vi "cooling.vi"() -> ()   [LabVIEW 2015]
panel:
  out "Output file path":path
  in  "Thick_max":bool[](array[boolean])=[FALSE, FALSE, FALSE, FALSE, FALSE, FALSE, FALSE, FALSE, FALSE, FALSE]
  in  "Thick_min":bool[](array[boolean])=[FALSE, FALSE, FALSE, FALSE, FALSE, FALSE, FALSE, FALSE, FALSE, FALSE]
  in  "Wid_max":bool[](array[boolean])=[FALSE, FALSE, FALSE, FALSE, FALSE, FALSE, FALSE, FALSE, FALSE, FALSE]
  in  "Apri database":bool
  in  "Insert IDs":bool
  in  "Stop Button":bool
  in  "Refresh Button":bool
  in  "Crea file di testo":bool
  in  "Wid_min":bool[](array[boolean])=[FALSE, FALSE, FALSE, FALSE, FALSE, FALSE, FALSE, FALSE, FALSE, FALSE]
  out "Bar name":string[](array[string])
  # "Cooling \"go - no go\" test"
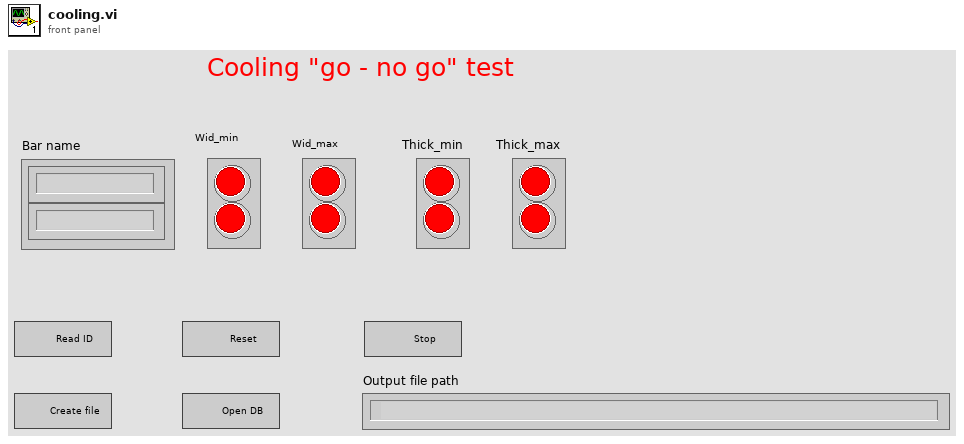
[diagram p1: front panel]
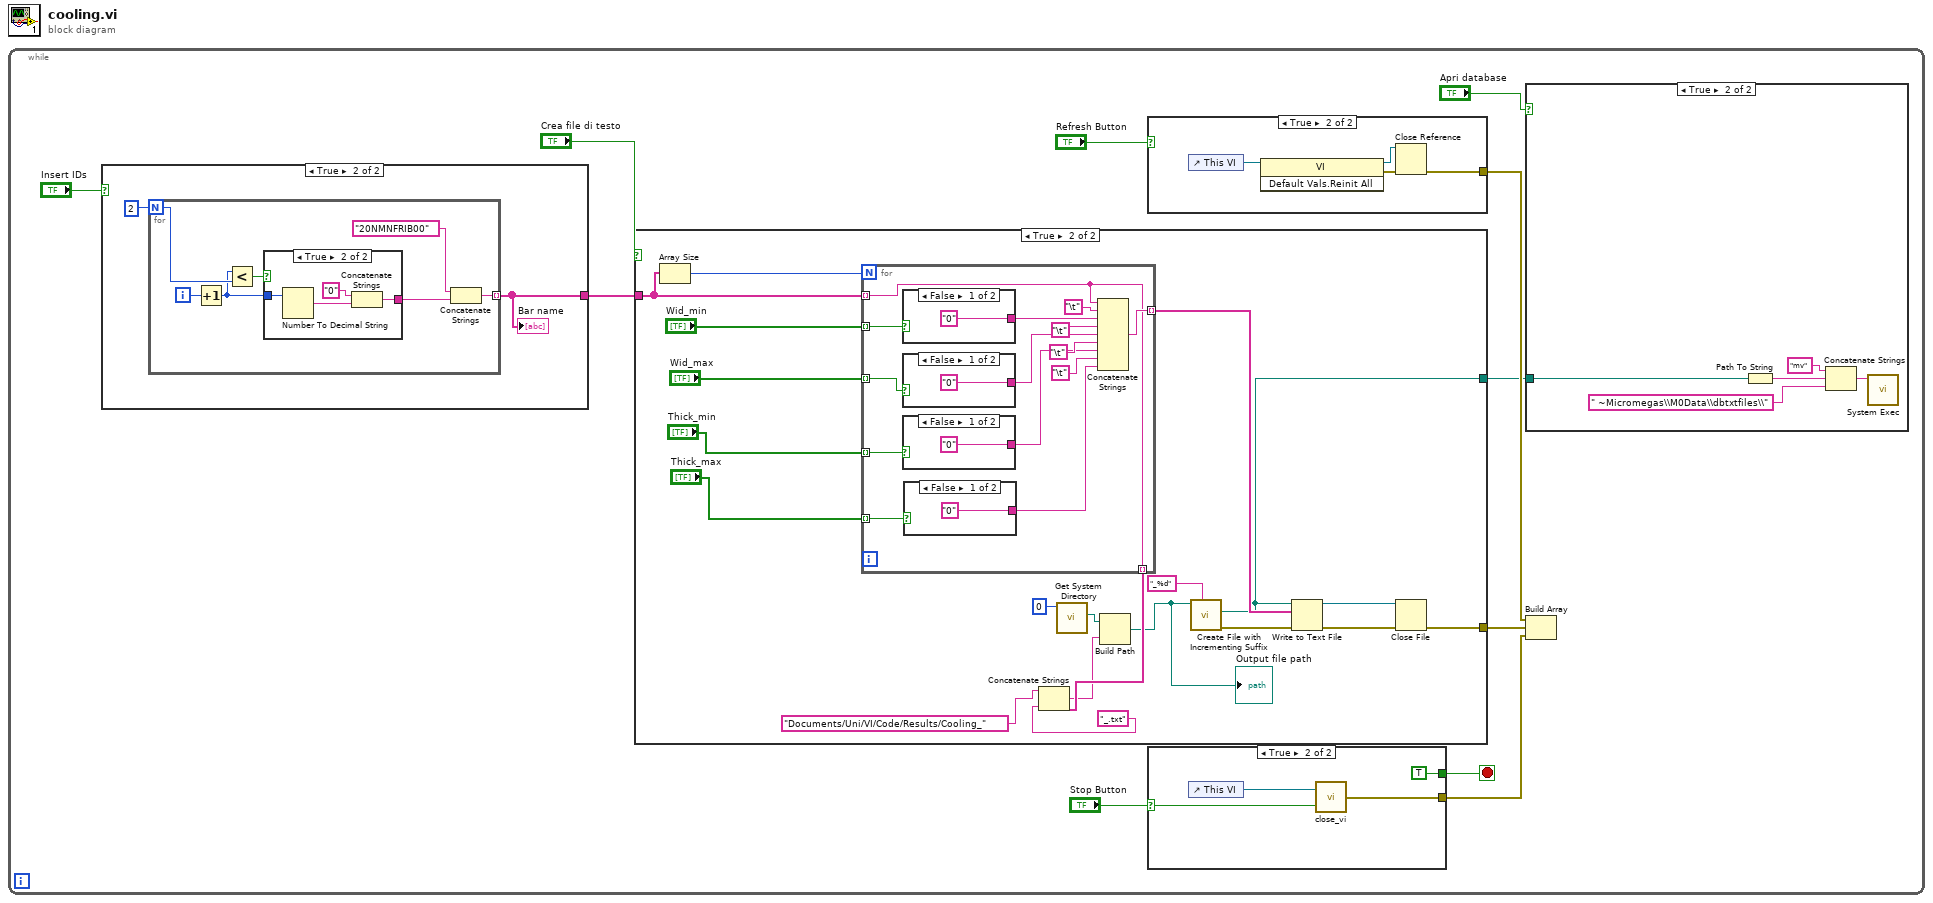
[diagram p0: block diagram]
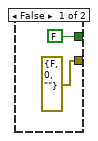
[diagram p3: hidden frame]
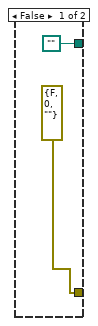
[diagram p4: hidden frame]
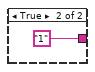
[diagram p5: hidden frame]
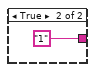
[diagram p6: hidden frame]
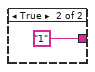
[diagram p7: hidden frame]
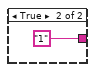
[diagram p8: hidden frame]
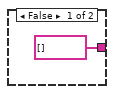
[diagram p9: hidden frame]
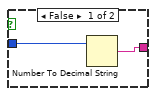
[diagram p10: hidden frame]
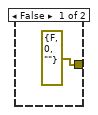
[diagram p11: hidden frame]
diagram:
  n1 = while {
    stop <- w3 stop-if-true
    n2 = case shown="True" "Insert IDs" {
      tunnel: [string[] [] w68] -> w8
      frame False {
      }
      frame True {
        n3 = for {
          N: 2 -> [w75]
          tunnel: [w70] -> w68 mode=indexing
          i -> [w74]
          n4 = Increment(x=w74) -> (x+1=w72:i32)
          n5 = Less?(x=w72, y=w75) -> (x < y?=w76:bool)
          n6 = case shown="True" w76 {
            tunnel: w72 -> [w78 w81]
            tunnel: [w77 w79] -> w71
            frame False {
              n7 = Number To Decimal String(number=w78) -> (decimal integer string=w77:string)  [unwired: 1 in]
            }
            frame True {
              n8 = Number To Decimal String(number=w81) -> (decimal integer string=w80:string)  [unwired: 1 in]
              n9 = Concatenate Strings("0", w80) -> (w79:string)
            }
          }
          n10 = Concatenate Strings("20NMNFRIB00", w71) -> (w70:string)
        }
        "Bar name" <- w68
      }
    }
    n11 = case shown="True" "Crea file di testo" {
      tunnel: w8 -> [_ w43]
      tunnel: [errorcluster {"status"=FALSE, "code"=0, "source"=""} ("error out") w36] -> w7
      tunnel: [path "" ("actual path") w35] -> w1
      frame False {
      }
      frame True {
        n12 = Array Size(array=w43) -> (size(s)=w44:i32)
        n13 = for {
          N: w44 -> [_]
          tunnel: w43 -> [w45] mode=indexing
          tunnel: "Wid_min" -> [w58] mode=indexing
          tunnel: [w55] -> w41 mode=indexing
          tunnel: "Wid_max" -> [w54] mode=indexing
          tunnel: "Thick_min" -> [w53] mode=indexing
          tunnel: "Thick_max" -> [w52] mode=indexing
          tunnel: [w45] -> w28 mode=indexing
          n14 = case shown="False" w58 {
            tunnel: ["0" "1"] -> w56
            frame False {
            }
            frame True {
            }
          }
          n15 = case shown="False" w54 {
            tunnel: ["0" "1"] -> w50
            frame False {
            }
            frame True {
            }
          }
          n16 = case shown="False" w53 {
            tunnel: ["0" "1"] -> w48
            frame False {
            }
            frame True {
            }
          }
          n17 = case shown="False" w52 {
            tunnel: ["0" "1"] -> w46
            frame False {
            }
            frame True {
            }
          }
          n18 = Concatenate Strings(w45, "\t", w56, "\t", w50, "\t", w48, "\t", w46) -> (w55:string)
        }
        n19 = Concatenate Strings("Documents/Uni/VI/Code/Results/Cooling_", w28, "_.txt") -> (w27:string)
        n20 = call <vilib>:"Get System Directory.vi"("system directory type"=0) -> ("system directory"=w30:path)  [unwired: 10 in]
        n21 = Build Path(base path=w30, name or relative path=w27) -> (appended path=w25:path)
        "Output file path" <- w25
        n22 = call <vilib>:"Create File with Incrementing Suffix.vi"("format string (\" (%d)\")"="_%d" ("format string (\" (%d)\")"), "file path"=w25) -> ("error out"=w40:errorcluster, "actual path"=w35:path)  [unwired: 7 in, 1 out]
        n23 = Write to Text File(file (use dialog)=w35, text=w41, error in=w40) -> (refnum out=w38:refnum<file>, error out=w39:errorcluster)  [unwired: 1 in, 1 out]
        n24 = Close File(refnum=w38, error in=w39) -> (error out=w36:errorcluster)  [unwired: 1 out]
      }
    }
    n25 = case shown="True" "Refresh Button" {
      tunnel: [errorcluster {"status"=FALSE, "code"=0, "source"=""} ("error out") w84] -> w5
      frame False {
      }
      frame True {
        n26 = control-ref of="This VI"() -> (w87:refnum<vi>)
        n27 = invoke class="VI" method="Default Vals.Reinit All"(reference=w87) -> (reference out=w86:refnum<vi>, error out=w85:errorcluster)  [unwired: 2 in, 1 out]
        n28 = Close Reference(reference=w86, error in (no error)=w85) -> (error out=w84:errorcluster)
      }
    }
    n29 = case shown="True" "Stop Button" {
      selector: "Stop Button" -> [_ w21]
      tunnel: [errorcluster {"status"=FALSE, "code"=0, "source"=""} ("error out") w22] -> w6
      tunnel: [FALSE TRUE] -> w3
      frame False {
      }
      frame True {
        n30 = control-ref of="This VI"() -> (w19:refnum<vi>)
        n31 = call "close_vi.vi"("Process Stop Button"=w21, "reference"=w19) -> ("error out"=w22:errorcluster)
      }
    }
    n32 = case shown="True" "Apri database" {
      tunnel: w1 -> [_ w16]
      frame False {
      }
      frame True {
        n33 = Path To String(path=w16) -> (string=w13:string)
        n34 = Concatenate Strings("mv" ("File Path Control"), w13, " ~Micromegas\\M0Data\\dbtxtfiles\\" ("string")) -> (w15:string)
        n35 = call <vilib>:"System Exec.vi"("command line"=w15) -> ()  [unwired: 7 in, 4 out]
      }
    }
    n36 = Build Array(w5, w7, w6) -> ()  [unwired: 1 out]
  }
